vi "Configure Math.vi"(0 "VISA resource name":refnum<visa-resource-name>, 1 "Function (0: Volts)":u16(ring) items=["Volts", "Current", "Resistance", "Digitize Voltage", "Digitize Current"], 2 "Math Operation (1: Percent)":u16(ring)=1 items=["Y= mx+b", "Percent", "Reciprocal"], 3 "M Value (1)":dbl=1.0, 4 "B Value (0)":dbl, 5 "error in (no error)":errorcluster, 6 "Enable Math Function (T:Disable)":bool=TRUE, 7 "Percent Value (1)":dbl=1.0) -> (14 "VISA resource name out":refnum<visa-resource-name>, 19 "error out":errorcluster)   [LabVIEW 2017, in "Keithley 2450.lvlib"]
doc: "Configure the math operation performed by the instrument on collected data."
uses:
  Keithley 2450.lvlib
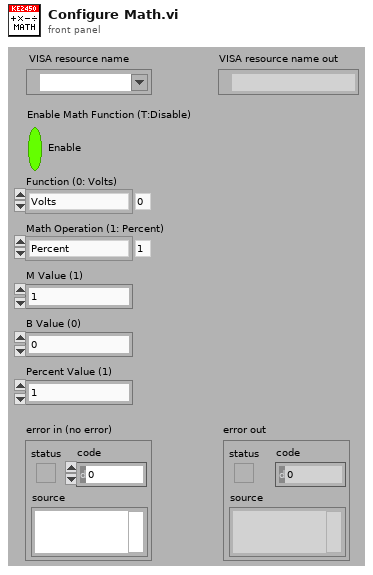
[diagram p1: front panel]
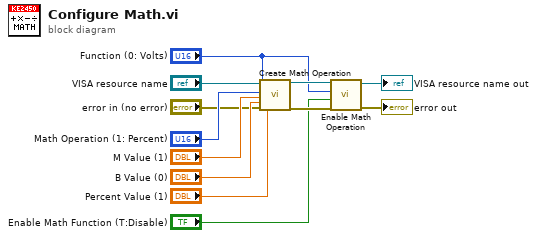
[diagram p0: block diagram]
diagram:
  n1 = call "Create Math Operation.vi"("VISA resource name"="VISA resource name", "Function (0: Volts)"="Function (0: Volts)", "Math Operation (1: Percent)"="Math Operation (1: Percent)", "M Value (0)"="M Value (1)", "B Value (1)"="B Value (0)", "error in (no error)"="error in (no error)", "Percent Value (1)"="Percent Value (1)") -> ("VISA resource name out"=w12:refnum<visa-resource-name>, "error out"=w11:errorcluster)  [unwired: 11 in]
  n2 = call "Enable Math Operation.vi"("error in (no error)"=w11, "Enable Math Operations (T:Enable)"="Enable Math Function (T:Disable)", "Function (0: Volts)"="Function (0: Volts)", "VISA resource name"=w12) -> ("error out"=→"error out":errorcluster, "VISA resource name out"=→"VISA resource name out":refnum<visa-resource-name>)  [unwired: 6 in]
